vi "Initalize connection.vi"() -> ()   [LabVIEW 2021, in "F-70 driver.lvlib"]
uses:
  F-70 driver.lvlib
  <vilib>/Instr/_visa.llb/VISA Configure Serial Port (Instr).vi
  <vilib>/ErrorRing/Error Ring.xnode
  <vilib>/Utility/error.llb/Error Cluster From Error Code.vi
panel:
  out "CRC-16":string
  out "elapsed hours":dbl
  out "revision":dbl
  out "error out":errorcluster
  in  "timeout (5s)":u32=5000
  in  "VISA resource name":refnum<visa-resource-name>="COM4"
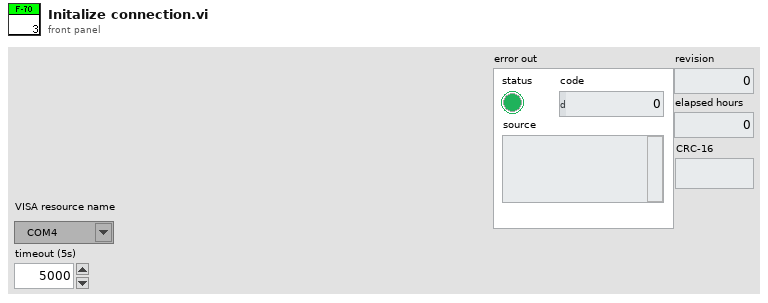
[diagram p1: front panel]
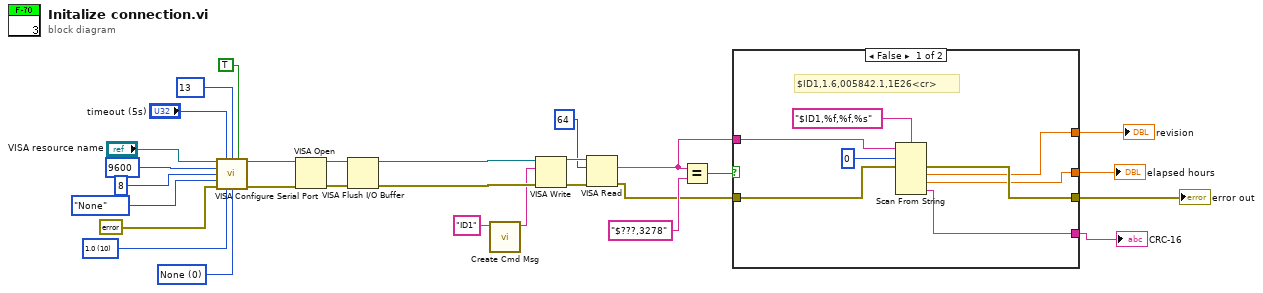
[diagram p0: block diagram]
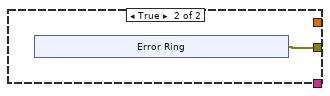
[diagram p2: hidden frame]
diagram:
  w29 = u16 0 items=["None", "XON/XOFF", "RTS/CTS", "XON/XOFF & RTS/CTS", "DTR/DSR", "XON/XOFF & DTR/DSR"] ("flow control (0:none)")
  w25 = u16 10 items=["1.0"=10, "1.5"=15, "2.0"=20] ("stop bits (10: 1 bit)")
  n1 = call-poly "VISA Configure Serial Port"("VISA resource name"="VISA resource name", "timeout (10sec)"="timeout (5s)", "termination char\n(0xA = '\\n' = LF)"=u8 13 ("termination char\n(0xA = '\\n' = LF)"), "Enable Termination\nChar (T)"=TRUE ("Enable Termination\nChar (T)"), "baud rate (9600)"=u32 9600, "data bits (8)"=u16 8, "parity (0:none)"=enum16{"None", "Odd", "Even", "Mark", "Space"}."None", "error in (no error)"=errorcluster {"status"=FALSE, "code"=0, "source"=""}, "stop bits (10: 1 bit)"=w25, "flow control (0:none)"=w29) -> ("VISA resource name out"=w19:refnum<visa-resource-name>, "error out"=w18:errorcluster)  [unwired: 4 in]
  n2 = VISA Open(error in (no error)=w18, VISA resource name=w19) -> (VISA resource name=w13:refnum<visa-resource-name>, error out=w12:errorcluster)  [unwired: 3 in]
  n3 = VISA Flush I/O Buffer(VISA resource name=w13, error in (no error)=w12) -> (VISA resource name out=w14:refnum<visa-resource-name>, error out=w17:errorcluster)  [unwired: 1 in]
  n4 = call "Create Cmd Msg.vi"("command"="ID1") -> ("complete message"=w11:string)  [unwired: 10 in]
  n5 = VISA Write(VISA resource name=w14, write buffer=w11, error in (no error)=w17) -> (VISA resource name out=w16:refnum<visa-resource-name>, error out=w15:errorcluster)  [unwired: 1 out]
  n6 = VISA Read(VISA resource name=w16, byte count=u32 64, error in (no error)=w15) -> (read buffer=w7:string, error out=w6:errorcluster)  [unwired: 2 out]
  n7 = Equal?(x=w7, y="$???,3278") -> (x = y?=w8:bool)
  n8 = case shown="False" w8 {
    tunnel: w7 -> [w31 _]
    tunnel: w6 -> [w36 _]
    tunnel: [w35 w38] -> w5
    tunnel: [w34 _] -> w4
    tunnel: [w33 _] -> w3
    tunnel: [w32 _] -> w2
    frame False {
      # "$ID1,1.6,005842.1,1E26<cr>"
      n9 = Scan From String(format string="$ID1,%f,%f,%s", input string=w31, initial scan location=u32 0, error in=w36) -> (error out=w35:errorcluster, output 1=w34:dbl, output 2=w33:dbl, output 3=w32:string)  [unwired: 3 in, 2 out]
    }
    frame True {
      n10 = xnode "Error Ring"() -> ("error out"=w38:errorcluster)
    }
  }
  "error out" <- w5
  "revision" <- w4
  "elapsed hours" <- w3
  "CRC-16" <- w2
